vi "Detect Zero Crossing pt by pt.vi"(7 "initialize":bool, 9 "direction (either)":enum16{"either", "minus-plus", "plus-minus"}(ring), 11 "input data point":dbl format="%0.2f") -> (3 "crossing":bool)   [LabVIEW 2015, in "Engine Simulation Toolkit System Explorer.lvlib"]
uses:
  Engine Simulation Toolkit System Explorer.lvlib
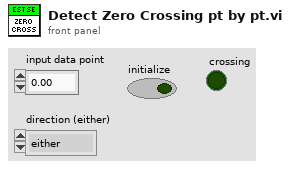
[diagram p1: front panel]
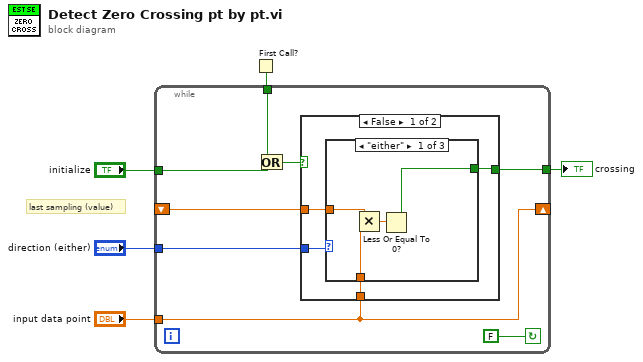
[diagram p0: block diagram]
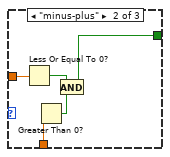
[diagram p2: hidden frame]
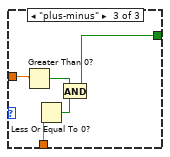
[diagram p3: hidden frame]
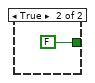
[diagram p4: hidden frame]
diagram:
  # "last sampling (value)"
  n1 = First Call?() -> (First Call?: T/F=w4:bool)
  n2 = while {
    tunnel: w4 -> [w9]
    tunnel: [w13] -> w5
    shift-left: _ -> [w12]
    shift-right: [w8] -> _
    tunnel: "input data point" -> [w8]
    tunnel: "initialize" -> [w7]
    tunnel: "direction (either)" -> [w6]
    stop <- FALSE continue-if-true
    n3 = Or(x=w9, y=w7) -> (x .or. y?=w10:bool)
    n4 = case shown="False" w10 {
      tunnel: [w14 FALSE] -> w13
      tunnel: w6 -> [w17 _]
      tunnel: w12 -> [w16 _]
      tunnel: w8 -> [w15 _]
      frame False {
        n5 = case shown="\"either\"" w17 {
          tunnel: w16 -> [w21 w26 w31]
          tunnel: w15 -> [w20 w25 w27]
          tunnel: [w18 w22 w28] -> w14
          frame "either" {
            n6 = Multiply(x=w21, y=w20) -> (x*y=w19:dbl)
            n7 = Less Or Equal To 0?(x=w19) -> (x <= 0?=w18:bool)
          }
          frame "minus-plus" {
            n8 = Less Or Equal To 0?(x=w26) -> (x <= 0?=w24:bool)
            n9 = Greater Than 0?(x=w25) -> (x > 0?=w23:bool)
            n10 = And(x=w24, y=w23) -> (x .and. y?=w22:bool)
          }
          frame "plus-minus" {
            n11 = Greater Than 0?(x=w31) -> (x > 0?=w30:bool)
            n12 = Less Or Equal To 0?(x=w27) -> (x <= 0?=w29:bool)
            n13 = And(x=w30, y=w29) -> (x .and. y?=w28:bool)
          }
        }
      }
      frame True {
      }
    }
  }
  "crossing" <- w5
